vi "fast_trigger_rising_edge_diag.vi"(8 "Second":bool, 10 "Ref_MLD measurement":dbl[][](array[numeric]), 11 "dt in":dbl) -> (3 "Waveform":waveform(dbl), 4 "First Rising edge index":i32, 6 "Frequency":dbl, 7 "Ref_MLD_triggered":dbl[][](array[numeric]))   [LabVIEW 2015]
uses:
  <vilib>/Analysis/baseanly.llb/Mean (DBL).vi
  <vilib>/Analysis/NI_AALBase.lvlib
panel:
  out "Waveform Graph 3":dbl[](graph)
  out "Waveform Graph 2":dbl[](graph)
  out "Waveform Graph":waveform(dbl)(graph)
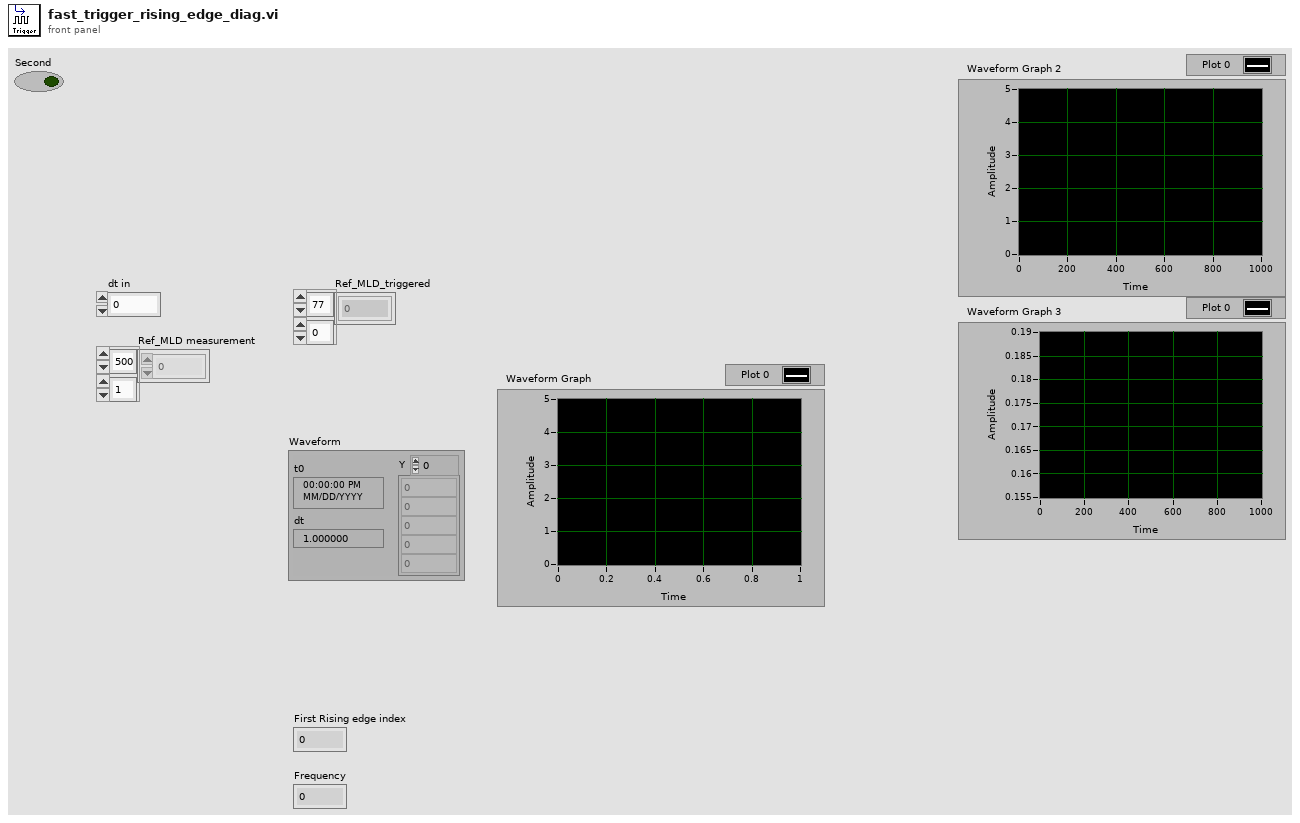
[diagram p1: front panel]
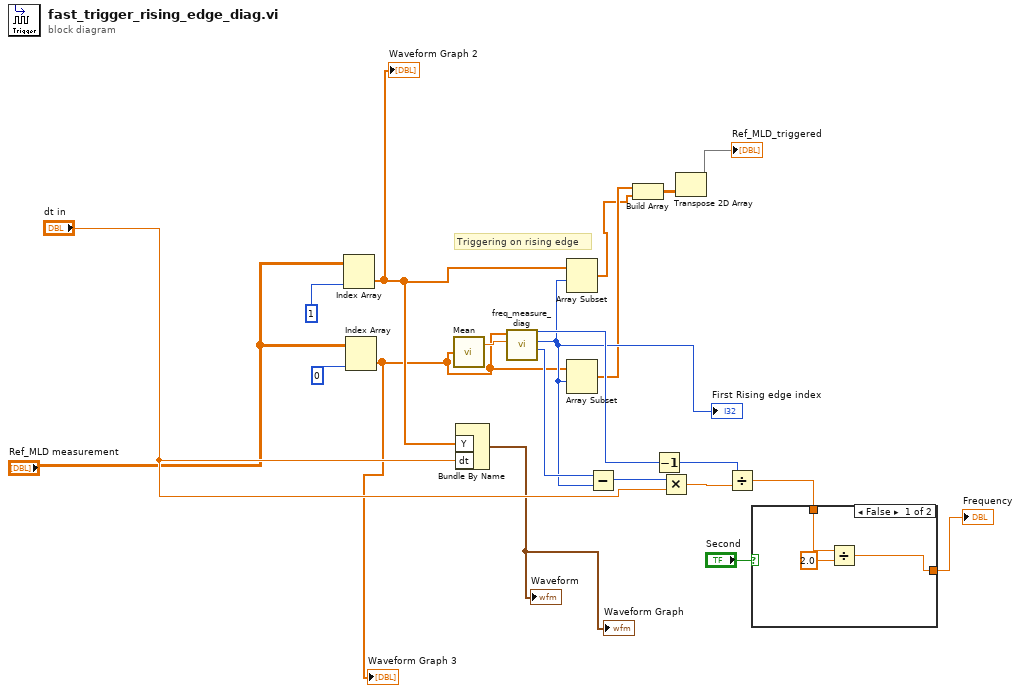
[diagram p0: block diagram]
diagram:
  # "Triggering on rising edge"
  n1 = Index Array(array="Ref_MLD measurement", index (col)=1 ("index (row)")) -> (element=w6:dbl[])  [unwired: 1 in]
  "Waveform Graph 2" <- w6
  n2 = Index Array(array="Ref_MLD measurement", index (col)=0 ("index (row)")) -> (element=w5:dbl[])  [unwired: 1 in]
  "Waveform Graph 3" <- w5
  n3 = call-poly <vilib>:"Mean.vi"("X"=w5) -> ("mean"=w17:dbl)  [unwired: 1 out]
  n4 = Bundle By Name("Y"=w6, "dt"="dt in") -> (→"Waveform" →"Waveform Graph":waveform(dbl))  [unwired: 1 in]
  n5 = call "freq_measure_diag.vi"("Ref_average"=w17, "data"=w5) -> ("Actual (last) Rising edge index"=w14:i32, "First Rising edge index"=w7:i32, "Rising edges"=w11:i32)  [unwired: 7 in]
  "First Rising edge index" <- w7
  n6 = Array Subset(array=w6, index=w7) -> (w3:dbl[])  [unwired: 1 in]
  n7 = Array Subset(array=w5, index=w7) -> (w4:dbl[])  [unwired: 1 in]
  n8 = Subtract(x=w14, y=w7) -> (x-y=w16:i32)
  n9 = Build Array(w4, w3) -> (w20:dbl[][])
  n10 = Decrement(x=w11) -> (x-1=w10:i32)
  n11 = Multiply(x=w16, y="dt in") -> (x*y=w15:dbl)
  n12 = Transpose 2D Array(2D array=w20) -> (transposed array=→"Ref_MLD_triggered":dbl[][])
  n13 = Divide(x=w10, y=w15) -> (x/y=w13:dbl)
  n14 = case shown="False" "Second" {
    tunnel: w13 -> [w24 w25]
    tunnel: [w22 w25] -> w2
    frame False {
      n15 = Divide(x=w24, y=2.0) -> (x/y=w22:dbl)
    }
    frame True {
    }
  }
  "Frequency" <- w2
